vi "Display Setup.vi"(0 "VISA resource name":refnum<visa-resource-name>, 1 "Enable Dots Only (F: Disable)":bool, 5 "Height (2: Large)":u16(ring)=2 items=["Small", "Medium", "Large"], 7 "Graticule Type (2: Full)":u16(ring)=2 items=["Crosshair", "Frame", "Full", "Grid"], 9 "Backlight (1: Medium)":u16(ring)=1 items=["Low", "Medium", "High"], 11 "error in (no error)":errorcluster, 12 "Graticule Visibility (50)":dbl=50.0, 13 "Waveform Visibility (70)":dbl=70.0) -> (4 "VISA resource name out":refnum<visa-resource-name>, 15 "error out":errorcluster)   [LabVIEW 2009, in "Tektronix DPO MSO 2000 4000 Series.lvlib"]
doc: "Sets the display settings of the oscilloscope."
uses:
  <instrlib>/Tektronix DPO MSO 2000 4000 Series/Tektronix DPO MSO 2000 4000 Series.lvlib
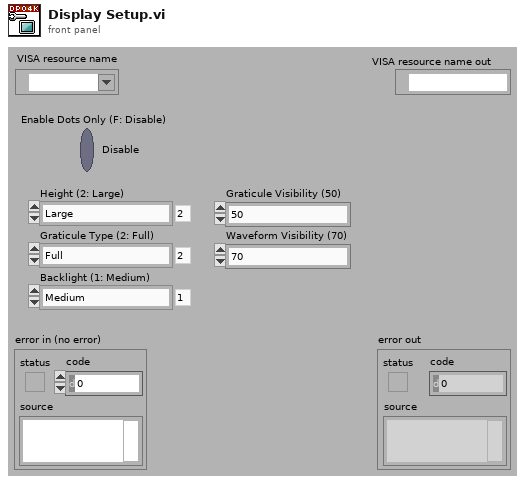
[diagram p1: front panel]
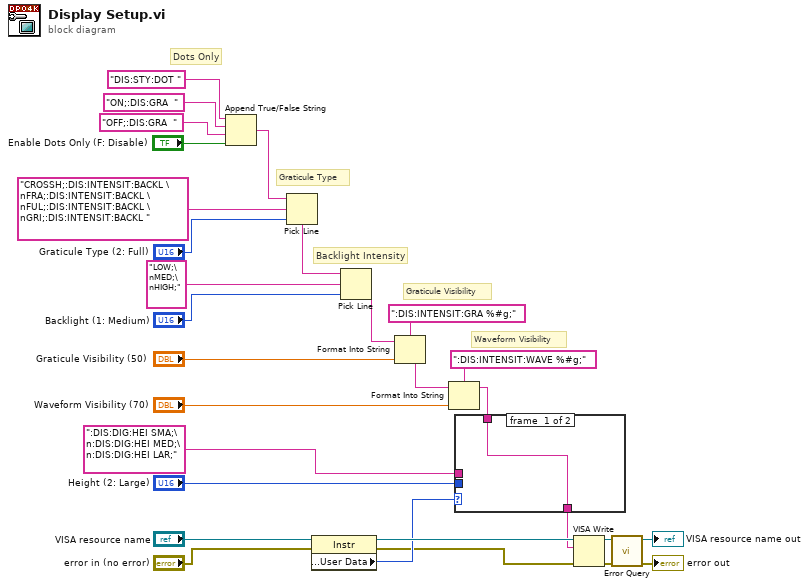
[diagram p0: block diagram]
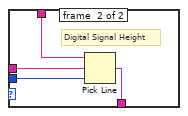
[diagram p2: hidden frame]
diagram:
  # "Waveform Visibility"
  # "Graticule Visibility"
  # "Backlight Intensity"
  # "Graticule Type"
  # "Dots Only"
  n1 = Append True/False String(1:"Enable Dots Only (F: Disable)", 2:"OFF;:DIS:GRA  " ("false string"), 3:"ON;:DIS:GRA  " ("true string"), 4:"DIS:STY:DOT ") -> (0:w10:string)
  n2 = Pick Line(string ("")=w10, multi-line string="CROSSH;:DIS:INTENSIT:BACKL \nFRA;:DIS:INTENSIT:BACKL \nFUL;:DIS:INTENSIT:BACKL \nGRI;:DIS:INTENSIT:BACKL ", line index="Graticule Type (2: Full)") -> (output string=w23:string)
  n3 = property class="Instr"(reference="VISA resource name", error in="error in (no error)") -> (reference out=w5:refnum<visa-resource-name>, error out=w2:errorcluster, "General Settings:User Data"=w4:u32)
  n4 = Pick Line(string ("")=w23, multi-line string="LOW;\nMED;\nHIGH;", line index="Backlight (1: Medium)") -> (output string=w20:string)
  n5 = Format Into String(format string=":DIS:INTENSIT:GRA %#g;", initial string=w20, "Graticule Visibility (50)") -> (resulting string=w17:string)  [unwired: 1 in, 1 out]
  n6 = Format Into String(format string=":DIS:INTENSIT:WAVE %#g;", initial string=w17, "Waveform Visibility (70)") -> (resulting string=w7:string)  [unwired: 1 in, 1 out]
  n7 = case shown="4..7, 14..19, 28..33" w4 {
    tunnel: "Height (2: Large)" -> [_ w34]
    tunnel: ":DIS:DIG:HEI SMA;\n:DIS:DIG:HEI MED;\n:DIS:DIG:HEI LAR;" ("multi-line string") -> [_ w33]
    tunnel: w7 -> [w30 w32]
    tunnel: [w30 w31] -> w1
    frame #0 {
    }
    frame #1 {
      # "Digital Signal Height"
      n8 = Pick Line(string ("")=w32, multi-line string=w33, line index=w34) -> (output string=w31:string)
    }
  }
  n9 = VISA Write(VISA resource name=w5, write buffer=w1, error in (no error)=w2) -> (VISA resource name out=w14:refnum<visa-resource-name>, error out=w13:errorcluster)  [unwired: 1 out]
  n10 = call <instrlib>:"Error Query.vi"("error in (no error)"=w13, "VISA resource name"=w14) -> ("error out"=→"error out":errorcluster, "VISA resource name out"=→"VISA resource name out":refnum<visa-resource-name>)  [unwired: 6 in, 2 out]
